vi "CSMSVMgr Sync to File.vi"(8 "error in (no error)":errorcluster, 11 "CSM-Static-Variable-Manager in":refnum<class "CSM-Static-Variable-Manager.lvclass">) -> (0 "error out":errorcluster, 3 "CSM-Static-Variable-Manager out":refnum<class "CSM-Static-Variable-Manager.lvclass">)   [LabVIEW 2017, in "INI-Static-Variable-Support.lvlib" / "CSM-Static-Variable-Manager.lvclass"]
uses:
  CSM-Static-Variable-Manager.lvclass
  CSM-Static-Variable-Manager.lvclass/CSM-Static-Variable-Manager.ctl
  LabVIEW-Config/Config.ctl
  LabVIEW-Config/LabVIEW-Config.lvlib
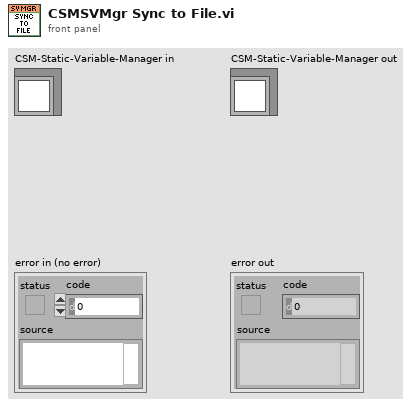
[diagram p1: front panel]
types:
  T1 = typedef "LabVIEW-Config.lvlib/Config.ctl" = cluster{"Path":path, "Lines":string[], "Tokens":enum8{"comment", "section", "key"}[], "Modified?":bool}
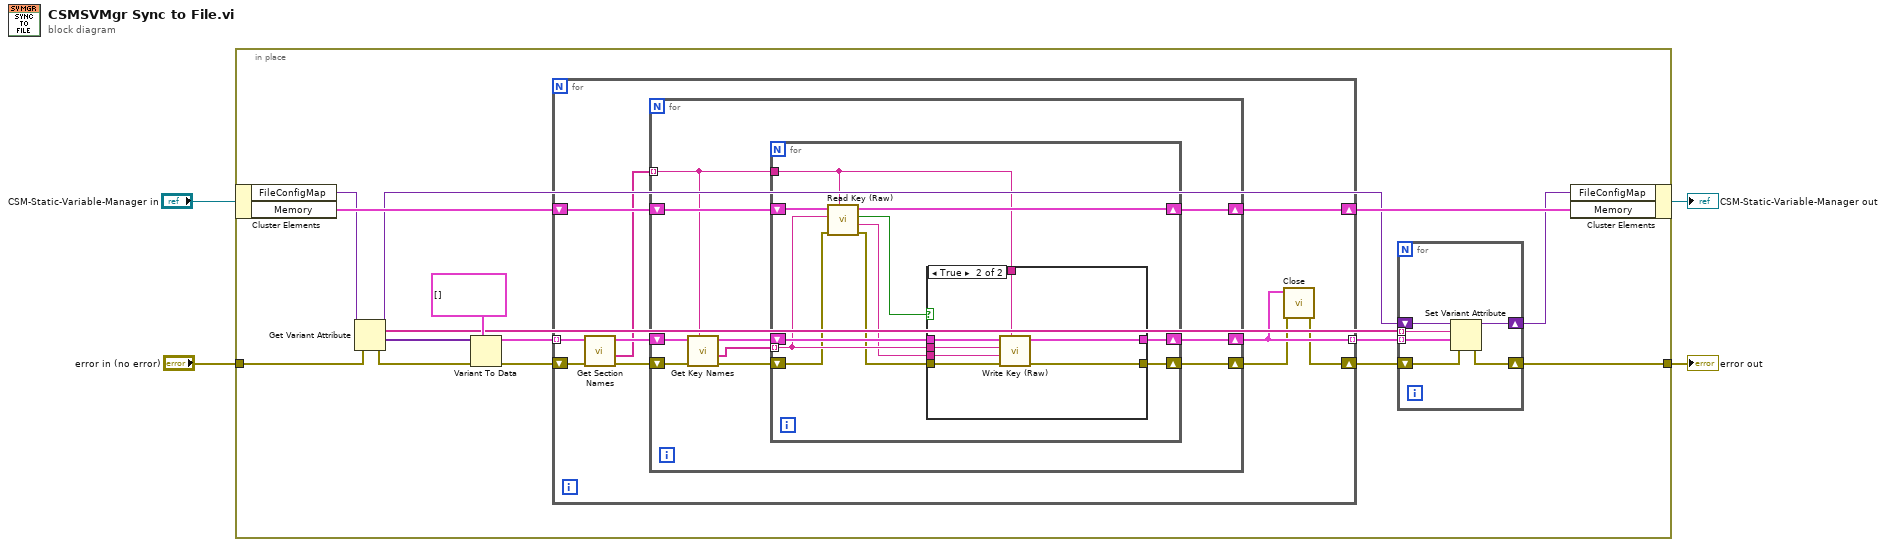
[diagram p0: block diagram]
diagram:
  n1 = in-place {
    in-place-border: "error in (no error)" -> [w14]
    in-place-border: [w10] -> w1
    n2 = in-place-cluster #1("CSM-Static-Variable-Manager in") -> ("FileConfigMap"=w17:variant, "Memory"=w19:T1)
    n3 = Get Variant Attribute(Variant=w17, error in=w14) -> (duplicate Variant=w8:variant, names=w5:string[], values=w16:variant[], error out=w15:errorcluster)  [unwired: 2 in]
    n4 = Variant To Data(error in=w15, type=T1[] [], Variant=w16) -> (data=w11:T1[], error out=w13:errorcluster)
    n5 = for {
      shift-right: [w33] -> w18
      shift-left: w19 -> [w34]
      shift-right: [w26] -> w9
      shift-left: w13 -> [w31]
      tunnel: w11 -> [w35] mode=indexing
      tunnel: [w28] -> w6 mode=indexing
      n6 = call "Get Section Names.vi"("error in (no error)"=w31, "Config in"=w35) -> ("error out"=w30:errorcluster, "Section Names"=w29:string[], "Config out"=w32:T1)  [unwired: 7 in]
      n7 = for {
        shift-right: [w41] -> w33
        shift-left: w34 -> [w42]
        shift-right: [w40] -> w27
        shift-left: w30 -> [w38]
        tunnel: w29 -> [w37] mode=indexing
        shift-right: [w36] -> w28
        shift-left: w32 -> [w39]
        n8 = call "Get Key Names.vi"("Section Name"=w37, "error in (no error)"=w38, "Config in"=w39) -> ("error out"=w43:errorcluster, "Key Names"=w44:string[], "Config out"=w45:T1)  [unwired: 5 in, 1 out]
        n9 = for {
          tunnel: w37 -> [w53]
          tunnel: w44 -> [w52] mode=indexing
          shift-right: [w50] -> w40
          shift-left: w43 -> [w51]
          shift-right: [w55] -> w41
          shift-left: w42 -> [w54]
          shift-right: [w49] -> w36
          shift-left: w45 -> [w56]
          n10 = call "Read Key (Raw).vi"("Section Name"=w53, "error in (no error)"=w51, "Key Name"=w52, "Config in"=w54) -> ("error out"=w46:errorcluster, "Content"=w47:string, "Key Found?"=w48:bool, "Config out"=w55:T1)  [unwired: 4 in]
          n11 = case shown="True" w48 {
            tunnel: w56 -> [w57 w65]
            tunnel: w53 -> [_ w64]
            tunnel: w52 -> [_ w63]
            tunnel: [w58 w62] -> w50
            tunnel: [w57 w61] -> w49
            tunnel: w47 -> [_ w60]
            tunnel: w46 -> [w58 w59]
            frame False {
            }
            frame True {
              n12 = call "Write Key (Raw).vi"("Section Name"=w64, "error in (no error)"=w59, "Content"=w60, "Key Name"=w63, "Config in"=w65) -> ("error out"=w62:errorcluster, "Config out"=w61:T1)  [unwired: 4 in, 1 out]
            }
          }
        }
      }
      n13 = call "Close.vi"("error in (no error)"=w27, "Config"=w28) -> ("error out"=w26:errorcluster)  [unwired: 8 in, 1 out]
    }
    n14 = for {
      shift-right: [w24] -> w10
      shift-left: w9 -> [w25]
      shift-right: [w22] -> w7
      shift-left: w8 -> [w23]
      tunnel: w6 -> [w21] mode=indexing
      tunnel: w5 -> [w20] mode=indexing
      n15 = Set Variant Attribute(Variant=w23, name=w20, value=w21, error in=w25) -> (Variant out=w22:variant, error out=w24:errorcluster)  [unwired: 1 out]
    }
    n16 = in-place-cluster #1("FileConfigMap"=w7, "Memory"=w18) -> (→"CSM-Static-Variable-Manager out":refnum<class "CSM-Static-Variable-Manager.lvclass">)
  }
  "error out" <- w1
